vi "CompVisionUtil_EstimateFieldToRobot_Alt.vi"(9 "CameraToRobot":T1={"TRANSLATION"={"X"=0.0, "Y"=0.0}, "ROTATION"={"VALUE"=0.0, "COS"=1.0, "SIN"=0.0}} {"ROTATION"."SIN" format="%13.4f"; "ROTATION"."COS" format="%13.4f"; "ROTATION"."VALUE" format="%13.4f"; "TRANSLATION"."Y" format="%14.3f"; "TRANSLATION"."X" format="%14.3f"}, 10 "FieldToTarget":T4={"TRANSLATION"={"X"=0.0, "Y"=0.0}, "ROTATION"={"VALUE"=0.0, "COS"=1.0, "SIN"=0.0}} {"ROTATION"."SIN" format="%13.4f"; "ROTATION"."COS" format="%13.4f"; "ROTATION"."VALUE" format="%13.4f"; "TRANSLATION"."Y" format="%14.3f"; "TRANSLATION"."X" format="%14.3f"}, 11 "CameraToTarget":T1={"TRANSLATION"={"X"=0.0, "Y"=0.0}, "ROTATION"={"VALUE"=0.0, "COS"=1.0, "SIN"=0.0}} {"ROTATION"."SIN" format="%13.4f"; "ROTATION"."COS" format="%13.4f"; "ROTATION"."VALUE" format="%13.4f"; "TRANSLATION"."Y" format="%14.3f"; "TRANSLATION"."X" format="%14.3f"}) -> (3 "EstimatedFieldToRobot":T1={"TRANSLATION"={"X"=0.0, "Y"=0.0}, "ROTATION"={"VALUE"=0.0, "COS"=1.0, "SIN"=0.0}} {"ROTATION"."SIN" format="%13.4f"; "ROTATION"."COS" format="%13.4f"; "ROTATION"."VALUE" format="%13.4f"; "TRANSLATION"."Y" format="%14.3f"; "TRANSLATION"."X" format="%14.3f"})   [LabVIEW 2019, in "Trajectory_Library.lvlib"]
doc: "Estimates the pose of the robot in the field coordinate system, given the position of the target relative to the camera, the target relative to the field, and the robot relative to the camera.\n\nInputs:\n -- CameraToTarget -- Transform containing the position of the target relative to the camera.\n -- FieldToTarget -- Pose containing the position of the target in the field.\n -- CameraToRobot -- Transform containing the position of the robot relative to the camera. If the camera was mounted 3 inches behind the \"origin\" (usually physical center) of the robot, this would be Transform2d(3 inches, 0 inches, 0 degrees).\n\nOutput:\n -- EstimatedCameraToTarget -- A Transform2d that takes us from the camera to the target.\n -- EstimatedFieldToRobot -- A Transform containing the position of the robot in the field."
uses:
  Trajectory_Library.lvlib
  TRANSLATION2D.ctl
  ROTATION2D.ctl
  POSE2D.ctl
  TRANSFORM2D.ctl
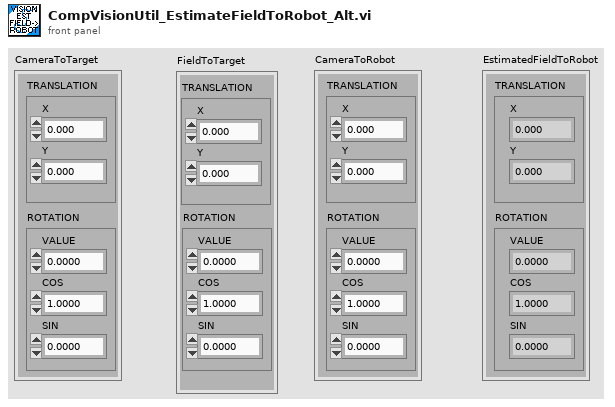
[diagram p1: front panel]
types:
  T1 = typedef "Trajectory_Library.lvlib/TRANSFORM2D.ctl" = cluster{"TRANSLATION":T2, "ROTATION":T3}
  T2 = typedef "Trajectory_Library.lvlib/TRANSLATION2D.ctl" = cluster{"X":dbl, "Y":dbl}
  T3 = typedef "Trajectory_Library.lvlib/ROTATION2D.ctl" = cluster{"VALUE":dbl, "COS":dbl, "SIN":dbl}
  T4 = typedef "Trajectory_Library.lvlib/POSE2D.ctl" = cluster{"TRANSLATION":T2, "ROTATION":T3}
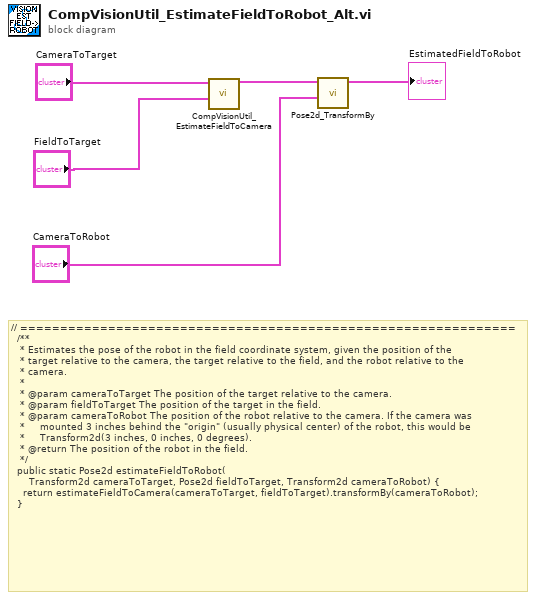
[diagram p0: block diagram]
diagram:
  # "// ==============================================================\n  /**\n   * Estimates the pose of the robot in the field coordinate system, given the position of the\n   * target relative to the camera, the target relative to the field, and the robot relative to the\n   * camera.\n   *\n   * @param cameraToTarget The position of the target relative to the camera.\n   * @param fieldToTarget The position of the target in the field.\n   * @param cameraToRobot The position of the robot relative to the camera. If the camera was\n   *     mounted 3 inches behind the \"origin\" (usually physical center) of the robot, this would be\n   *     Transform2d(3 inches, 0 inches, 0 degrees).\n   * @return The position of the robot in the field.\n   */\n  public static Pose2d estimateFieldToRobot(\n      Transform2d cameraToTarget, Pose2d fieldToTarget, Transform2d cameraToRobot) {\n    return estimateFieldToCamera(cameraToTarget, fieldToTarget).transformBy(cameraToRobot);\n  }"
  n1 = call "CompVisionUtil_EstimateFieldToCamera.vi"("FieldToTarget"="FieldToTarget", "CameraToTarget"="CameraToTarget") -> ("EstimateFieldToCamera"=w3:T4)  [unwired: 9 in]
  n2 = call "Pose2d_TransformBy.vi"("other TRANSFORM"="CameraToRobot", "in POSE"=w3) -> ("out POSE"=→"EstimatedFieldToRobot":T4)  [unwired: 9 in]
